vi "NumToBinWord.vi"(6 "# of bits":i16=3, 8 "error in (no error)":errorcluster, 10 "bin num":i32=1 min=0 max=1) -> (0 "error out":errorcluster, 2 "bin word (str)":string)   [LabVIEW 2018]
doc: "This vi will take in a number (usually trunciated by excel) and format ot it into a n Bit word. It is used for sending numbers into labview via excel and maintaining the word length.\n\nUse the \"# of bits\" to adjust the length of the output number"
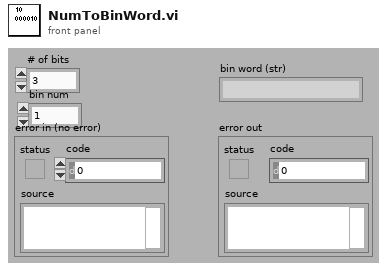
[diagram p1: front panel]
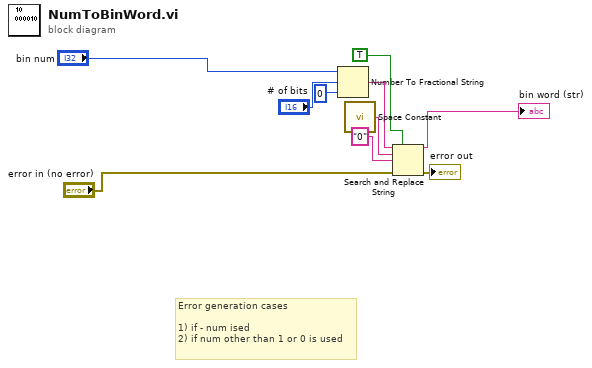
[diagram p0: block diagram]
diagram:
  # "Error generation cases\n\n1) if - num ised \n2) if num other than 1 or 0 is used"
  n1 = Number To Fractional String(number="bin num", width (-)="# of bits", precision (6)=i16 0) -> (F-format string=w8:string)  [unwired: 1 in]
  n2 = call <vilib>:"Space Constant.vi"() -> ("String"=w6:string)
  n3 = Search and Replace String(replace all?=TRUE ("replace all? (F)"), input string=w8, search string=w6, replace string="0" ("replace string (\"\")"), error in="error in (no error)") -> (result string=→"bin word (str)":string, error out=→"error out":errorcluster)  [unwired: 3 in, 2 out]
